vi "RT_TVA_DATA.vi"(11 "TVA_Data":u64[](array[numeric])) -> (0 "Dest address":u8, 1 "Souce address":u8, 2 "Yaw Angle":dbl(knob) scale=-3.0..3.0, 3 "Pitch Angle":dbl(knob) scale=-3.0..3.0, 4 "Data CRC Fault":bool, 6 "Address CRC Fault":bool)   [LabVIEW 2017]
panel:
  out "element":u64 format="%x"
  out "element 4":u64 format="%x"
  out "element 3":u64 format="%x"
  out "element 2":u64 format="%x"
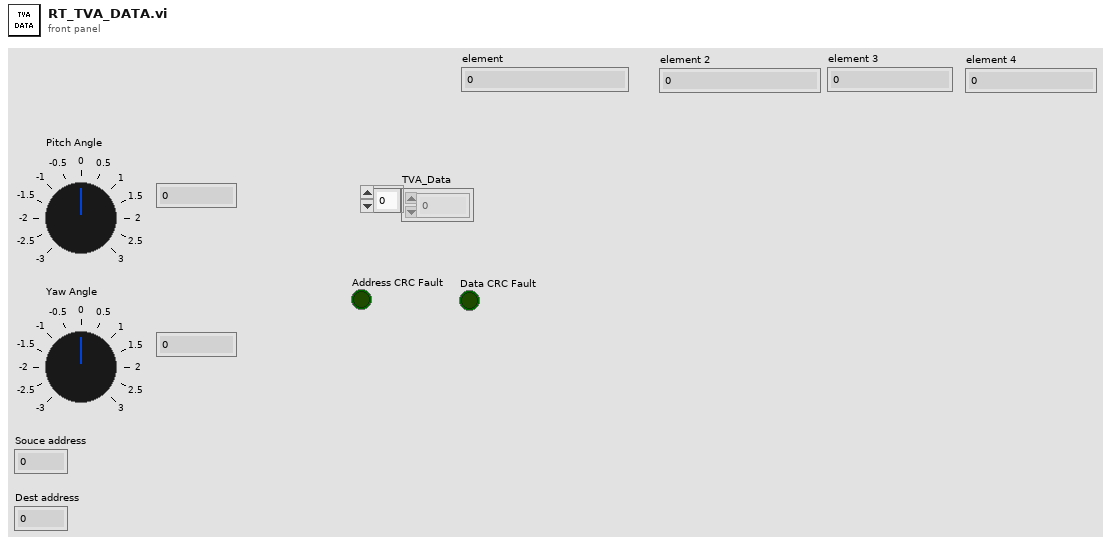
[diagram p1: front panel]
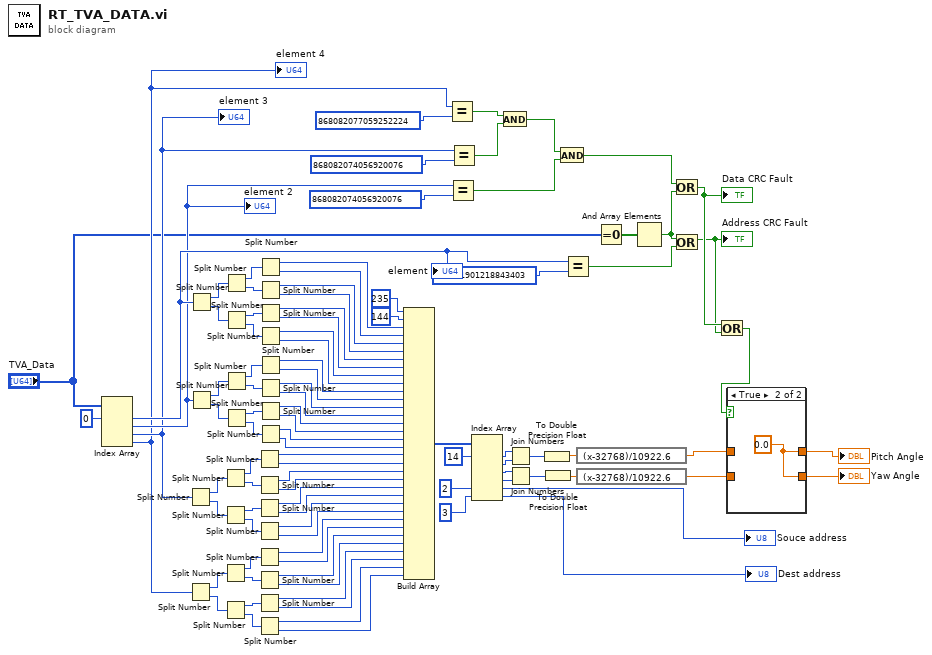
[diagram p0: block diagram]
diagram:
  n1 = Index Array(array="TVA_Data", index #1=0 ("index")) -> (element #1=w23:u64, element #2=w20:u64, element #3=w18:u64, element #4=w16:u64)  [unwired: 3 in]
  "element 2" <- w20
  "element 3" <- w18
  "element 4" <- w16
  "element" <- w23
  n2 = Split Number(x=w18) -> (hi(x)=w39:u32, lo(x)=w40:u32)
  n3 = Split Number(x=w16) -> (hi(x)=w50:u32, lo(x)=w49:u32)
  n4 = Split Number(x=w23) -> (hi(x)=w27:u32, lo(x)=w28:u32)
  n5 = Split Number(x=w20) -> (hi(x)=w38:u32, lo(x)=w37:u32)
  n6 = Split Number(x=w39) -> (hi(x)=w41:u16, lo(x)=w42:u16)
  n7 = Split Number(x=w40) -> (hi(x)=w43:u16, lo(x)=w44:u16)
  n8 = Split Number(x=w50) -> (hi(x)=w48:u16, lo(x)=w47:u16)
  n9 = Split Number(x=w49) -> (hi(x)=w46:u16, lo(x)=w45:u16)
  n10 = Split Number(x=w27) -> (hi(x)=w29:u16, lo(x)=w30:u16)
  n11 = Split Number(x=w28) -> (hi(x)=w31:u16, lo(x)=w32:u16)
  n12 = Split Number(x=w38) -> (hi(x)=w36:u16, lo(x)=w35:u16)
  n13 = Split Number(x=w37) -> (hi(x)=w34:u16, lo(x)=w33:u16)
  n14 = Split Number(x=w41) -> (hi(x)=w66:u8, lo(x)=w67:u8)
  n15 = Split Number(x=w42) -> (hi(x)=w68:u8, lo(x)=w69:u8)
  n16 = Split Number(x=w43) -> (hi(x)=w70:u8, lo(x)=w71:u8)
  n17 = Split Number(x=w44) -> (hi(x)=w72:u8, lo(x)=w73:u8)
  n18 = Split Number(x=w48) -> (hi(x)=w74:u8, lo(x)=w75:u8)
  n19 = Split Number(x=w47) -> (hi(x)=w76:u8, lo(x)=w77:u8)
  n20 = Split Number(x=w46) -> (hi(x)=w78:u8, lo(x)=w79:u8)
  n21 = Split Number(x=w45) -> (hi(x)=w96:u8, lo(x)=w97:u8)
  n22 = Split Number(x=w29) -> (hi(x)=w51:u8, lo(x)=w52:u8)
  n23 = Split Number(x=w30) -> (hi(x)=w53:u8, lo(x)=w54:u8)
  n24 = Split Number(x=w31) -> (hi(x)=w55:u8, lo(x)=w56:u8)
  n25 = Split Number(x=w32) -> (hi(x)=w57:u8, lo(x)=w58:u8)
  n26 = Split Number(x=w36) -> (hi(x)=w24:u8, lo(x)=w59:u8)
  n27 = Split Number(x=w35) -> (hi(x)=w60:u8, lo(x)=w61:u8)
  n28 = Split Number(x=w34) -> (hi(x)=w62:u8, lo(x)=w63:u8)
  n29 = Split Number(x=w33) -> (hi(x)=w64:u8, lo(x)=w65:u8)
  n30 = Build Array(u8 235 ("x"), u8 144 ("x"), w51, w52, w53, w54, w55, w56, w57, w58, w24, w59, w60, w61, w62, w63, w64, w65, w66, w67, w68, w69, w70, w71, w72, w73, w74, w75, w76, w77, w78, w79, w96, w97) -> (w80:u8[])
  n31 = Equal?(x=w16, y=u64 868082077059252224) -> (x = y?=w15:bool)
  n32 = Equal?(x=w20, y=u64 868082074056920076) -> (x = y?=w12:bool)
  n33 = Equal?(x=w18, y=u64 868082074056920076) -> (x = y?=w14:bool)
  n34 = Index Array(array=w80, index #1=14 ("index"), index #5=2 ("index"), index #6=3 ("index")) -> (element #1=w84:u8, element #2=w85:u8, element #3=w86:u8, element #4=w87:u8, element #5=→"Souce address":u8, element #6=→"Dest address":u8)  [unwired: 3 in]
  n35 = And(x=w15, y=w14) -> (x .and. y?=w13:bool)
  n36 = Join Numbers(hi=w84, lo=w85) -> ((hi.lo)=w89:u16)
  n37 = Join Numbers(hi=w86, lo=w87) -> ((hi.lo)=w88:u16)
  n38 = To Double Precision Float(number=w89) -> (double precision float=w91:dbl)
  n39 = To Double Precision Float(number=w88) -> (double precision float=w90:dbl)
  n40 = And(x=w13, y=w12) -> (x .and. y?=w8:bool)
  n41 = Equal?(x=w23, y=u64 795741901218843403) -> (x = y?=w22:bool)
  n42 = expression code="(x-32768)/10922.6"(w91) -> (w2:dbl)
  n43 = expression code="(x-32768)/10922.6"(w90) -> (w1:dbl)
  n44 = Equal To 0?(x="TVA_Data") -> (x = 0?=w10:bool[])
  n45 = And Array Elements(Boolean array=w10) -> (logical AND=w9:bool)
  n46 = Or(x=w8, y=w9) -> (x .or. y?=w7:bool)
  "Data CRC Fault" <- w7
  n47 = Or(x=w9, y=w22) -> (x .or. y?=w6:bool)
  "Address CRC Fault" <- w6
  n48 = Or(x=w7, y=w6) -> (x .or. y?=w5:bool)
  n49 = case shown="True" w5 {
    tunnel: [w99 w100] -> w4
    tunnel: [w98 w100] -> w3
    tunnel: w2 -> [w99 _]
    tunnel: w1 -> [w98 _]
    frame False {
    }
    frame True {
      w100 = 0.0
    }
  }
  "Yaw Angle" <- w3
  "Pitch Angle" <- w4
